vi "Event - Load Event Log.vi"(8 "error in":errorcluster) -> (0 "error out":errorcluster)   [LabVIEW 2019]
uses:
  Controls/Report - State.ctl
  Controls/Report - Data Structure.ctl
  <vilib>/httpClient/ClientHandle.ctl
  Controls/FGV States.ctl
  Controls/eFGV States.ctl
  Controls/JSON - Fileid.ctl
  <vilib>/httpClient/POSTBuffer.vi
  <vilib>/httpClient/LabVIEWHTTPClient.lvlib
panel:
  out "data":T1(array[cluster])
  in  "Tab Control":enum32{"Page 1", "Page 2"}(tab)
  in  "Listbox":i32(listbox)=-1 caption="Select Test"
  in  "Search":string
  in  "Generate":bool
  in  "Cancel":bool
  out "Total":u32
  in  "Pages":u32
  in  "Forward":bool
  in  "Back":bool
  in  "Event List":i32(listbox)
  in  "Back":bool
  # "of"
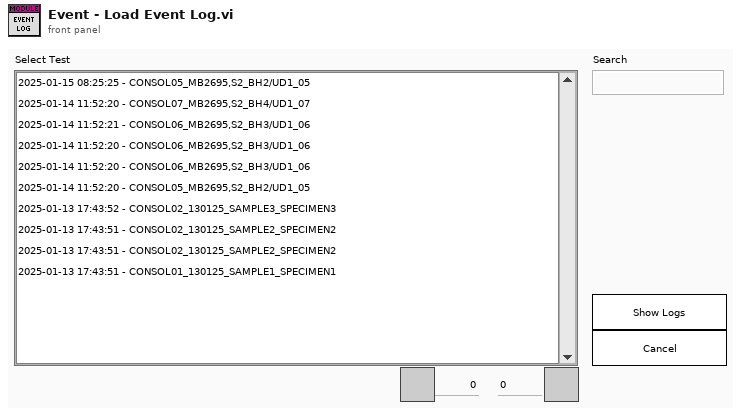
[diagram p1: front panel]
types:
  T1 = cluster{"id":string, "created_date":string, "testname":string, "jobno":string, "jobdesc":string, "sampleid":string, "date":string, "specimentno":string, "depth":string, "height":string, "diameter":string, "weight":string, "done":string}[]
  T2 = typedef "Report - State.ctl" = enum16{"Init", "Get File List", "Get Station Name", "Parse File List", "Idle", "Prepare to Generate", "Get Report", "Parse Report", "Get Data", "View T90", "Parse Data", "Convert to Excel", "Clean Up", "Close"}
  T3 = typedef "eFGV States.ctl" = enum16{"Init", "Read", "Write", "Exit"}
  T4 = typedef "FGV States.ctl" = enum16{"Read", "Write"}
  T5 = typedef "Report - Data Structure.ctl" = cluster{"API Ref":T6, "FileList":string[][], "Fileid":string, "testname":string[], "testtype":string[], "tdms":refnum<k34>, "TDMS Path":path, "tdms_path":string, "excel_path":string, "Excel Path":path, "List Name":string[], "Station Name":string[], "Plot":bool, "Tangent Point":string}
  T6 = typedef "LabVIEWHTTPClient.lvlib/ClientHandle.ctl" = refnum<k1>
  T7 = typedef "JSON - Fileid.ctl" = cluster{"status":string, "data":cluster{"id":string, "created_date":string, "testname":string, "jobno":string, "jobdesc":string, "sampleid":string, "date":string, "specimentno":string, "depth":string, "height":string, "diameter":string, "weight":string, "done":string}[]}
  T8 = cluster{"status":string, "data":cluster{"id":string, "created_date":string, "filename":string, "stage":string, "testplan":string, "station":string, "status":string, "delete":string}[]}
  T9 = cluster{"status":string, "data":cluster{"created_date":string, "message":string}[]}
  T10 = cluster{"id":string, "created_date":string, "filename":string, "stage":string, "testplan":string, "station":string, "status":string, "delete":string}[]
  T11 = cluster{"id":string, "created_date":string, "filename":string, "stage":string, "testplan":string, "station":string, "status":string, "delete":string}
  T12 = typedef "eventvkey.ctl" = enum16{"ASCII", "Enter", "Return", "Shift", "Ctrl", "Alt", "Cmd", "Opt", "Caps", "NumLock", "Clear", "Break", "Up", "Down", "Left", "Right", "Insert", "Delete", "Home", "End", "PageUp", "PageDown", "Escape", "Help", "Pause", "ScrollLock", "F1", "F2", "F3", "F4", "F5", "F6", "F7", "F8", "F9", "F10", "F11", "F12", "F13", "F14", "F15", "F16", "F17", "F18", "F19", "F20", "F21", "F22", "F23", "F24", "Play", "VolumeUp", "VolumeDown", "Mute", "Two Byte Char"}
  T13 = cluster{"created_date":string, "message":string}[]
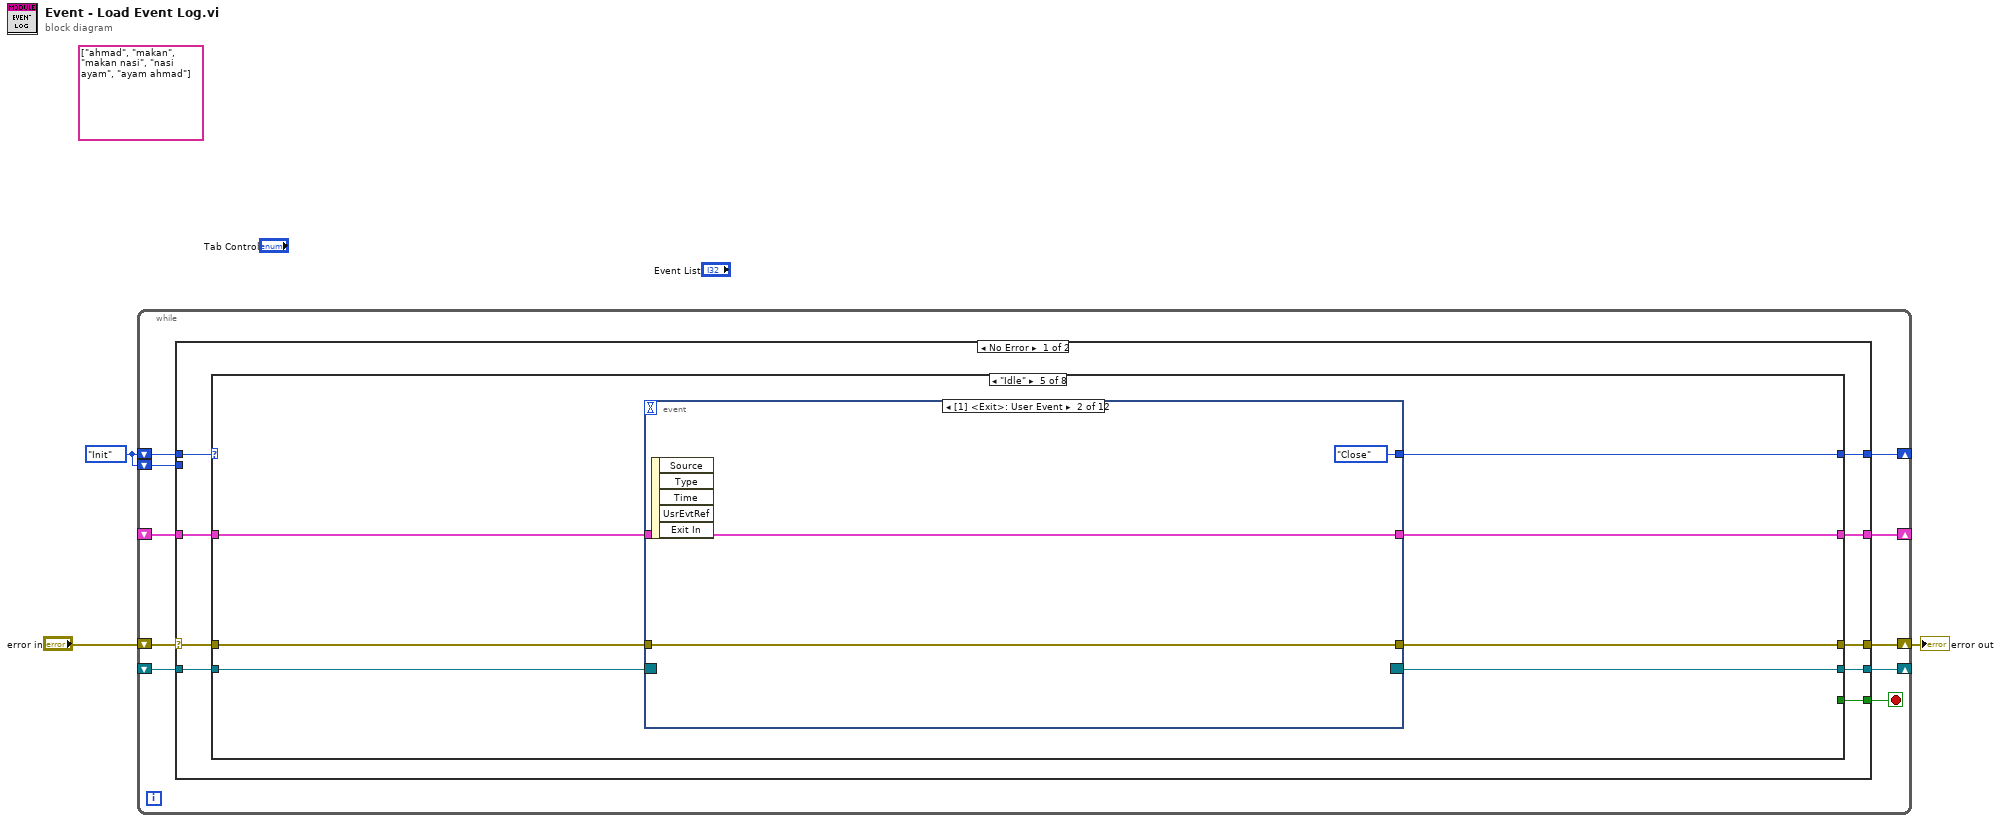
[diagram p0: block diagram]
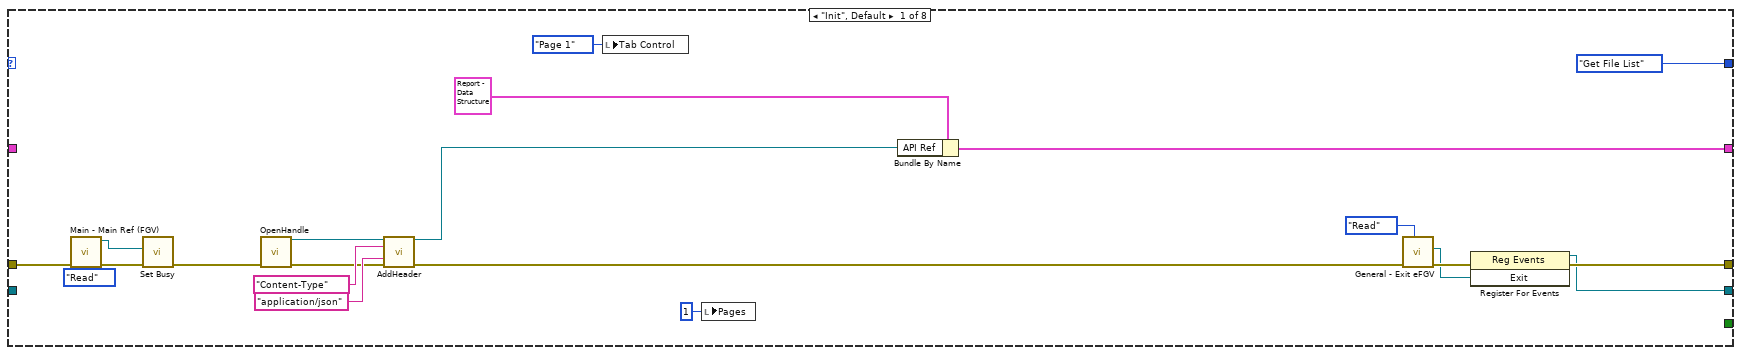
[diagram p2: hidden frame]
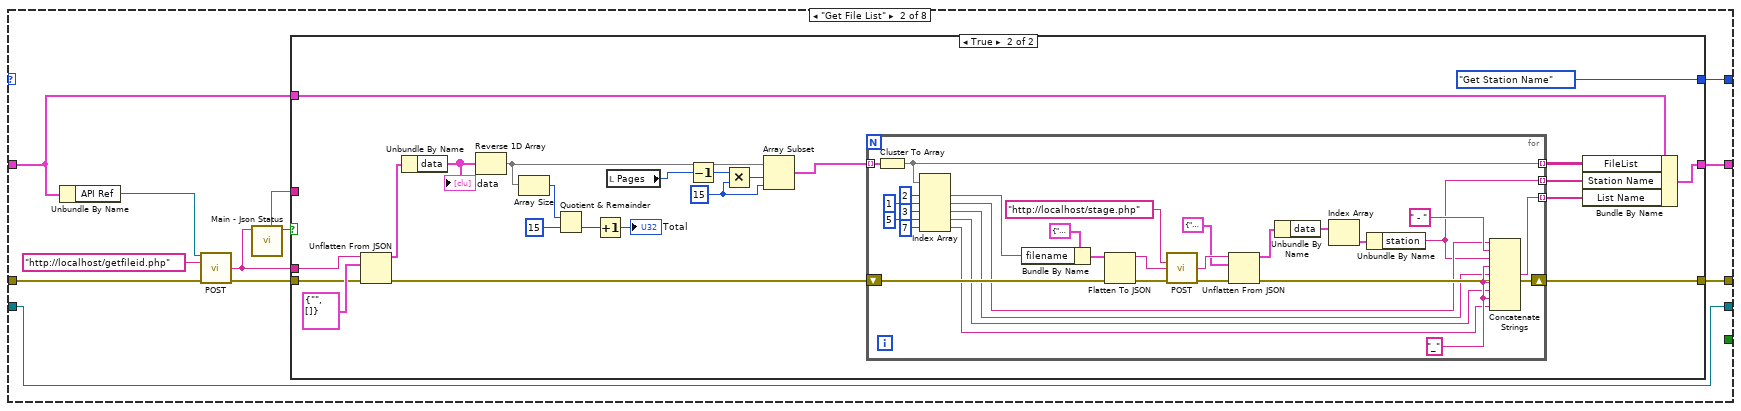
[diagram p3: hidden frame]
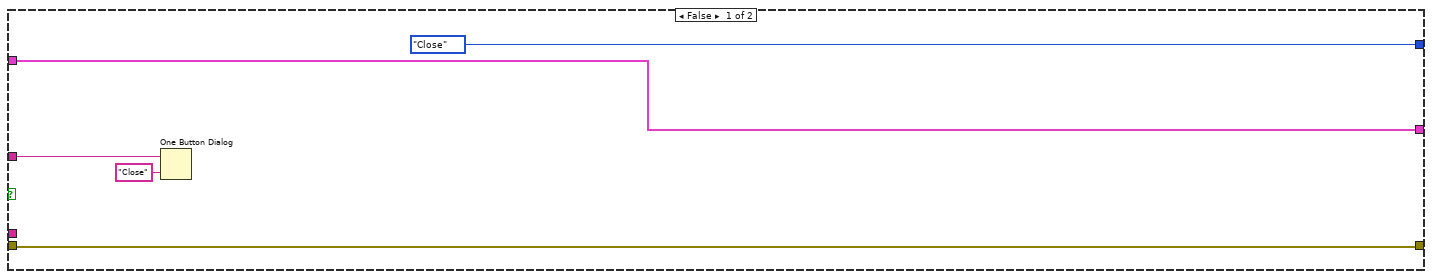
[diagram p4: hidden frame]
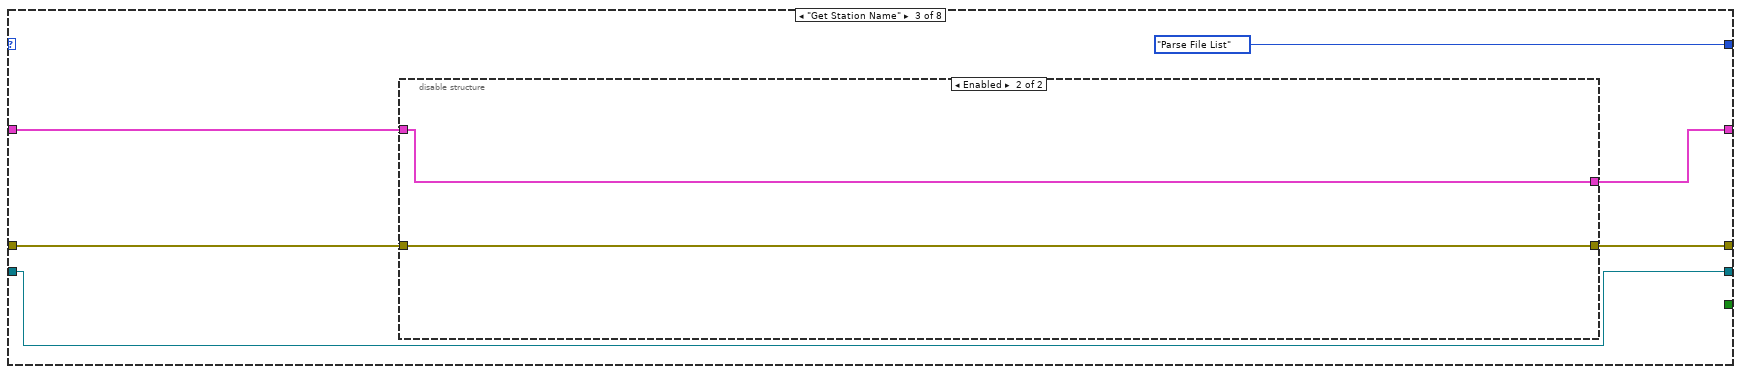
[diagram p5: hidden frame]
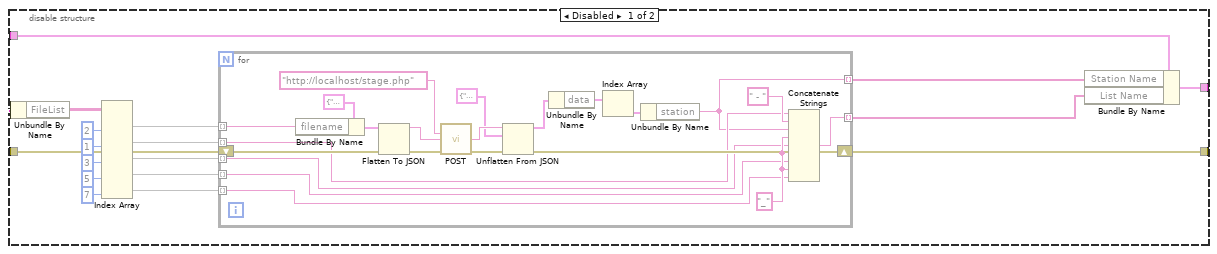
[diagram p6: hidden frame]
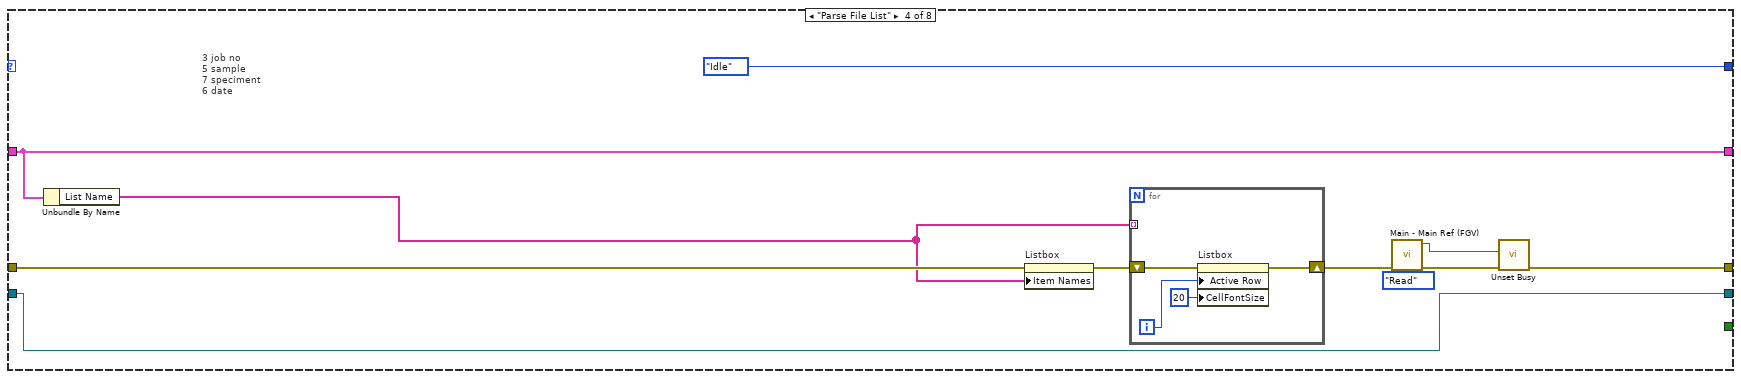
[diagram p7: hidden frame]
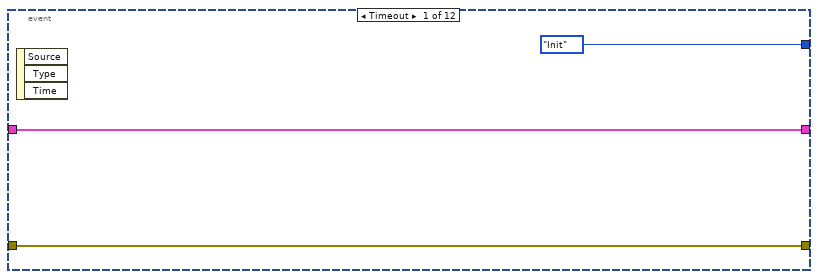
[diagram p8: hidden frame]
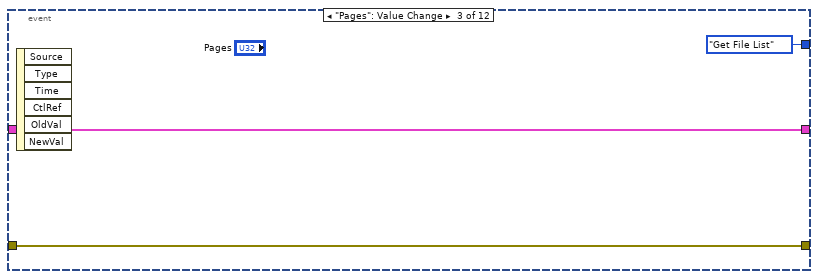
[diagram p9: hidden frame]
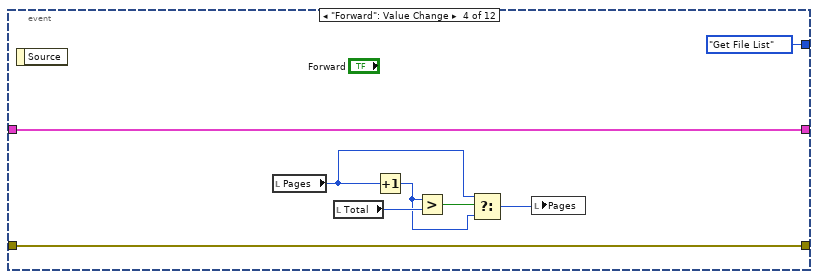
[diagram p10: hidden frame]
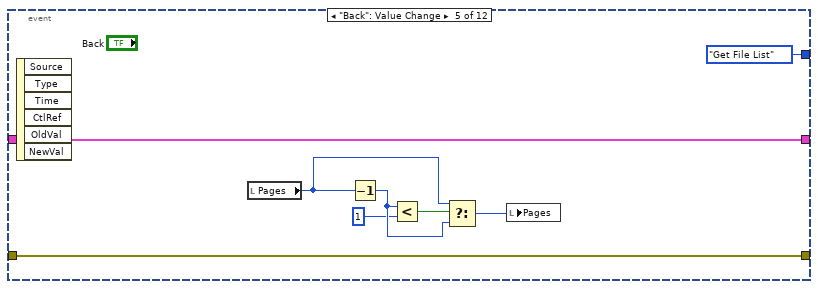
[diagram p11: hidden frame]
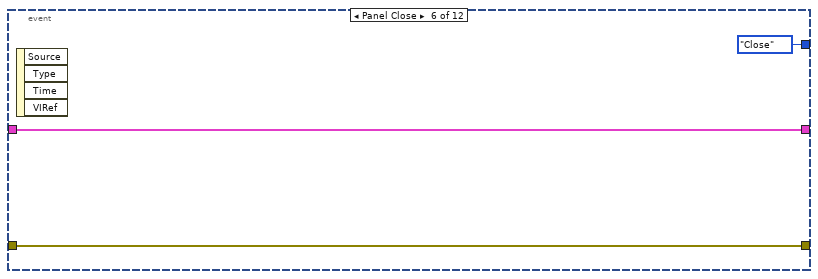
[diagram p12: hidden frame]
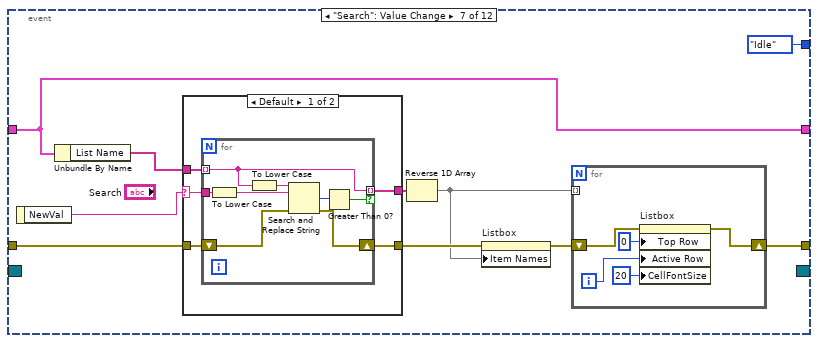
[diagram p13: hidden frame]
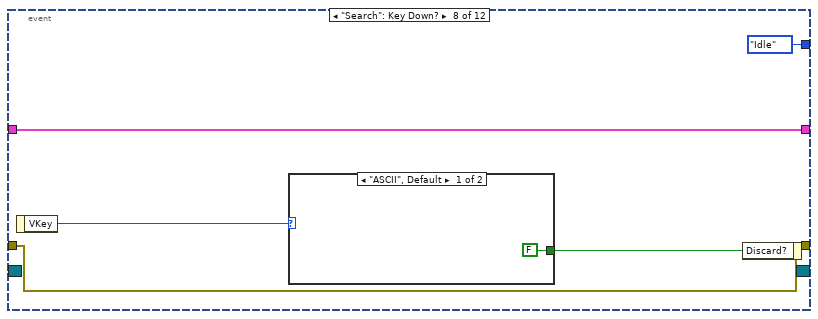
[diagram p15: hidden frame]
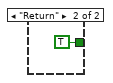
[diagram p16: hidden frame]
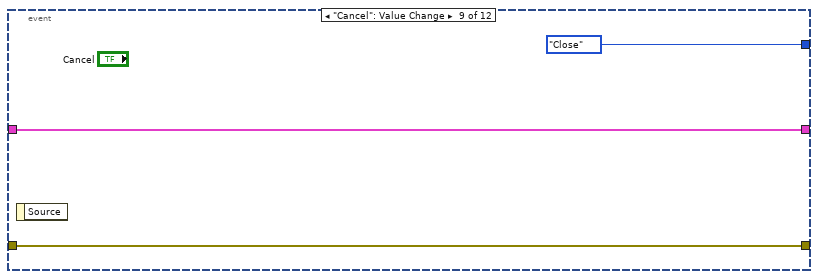
[diagram p17: hidden frame]
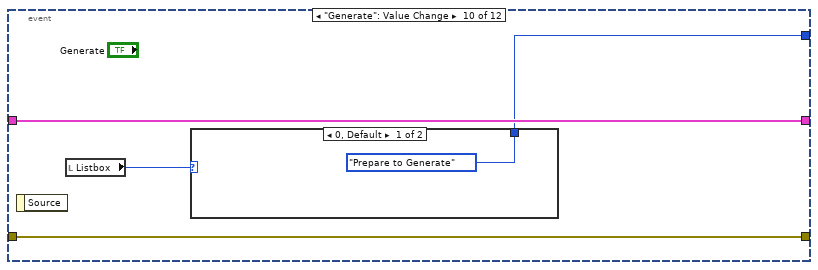
[diagram p18: hidden frame]
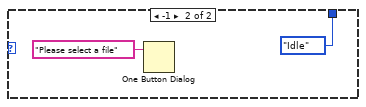
[diagram p19: hidden frame]
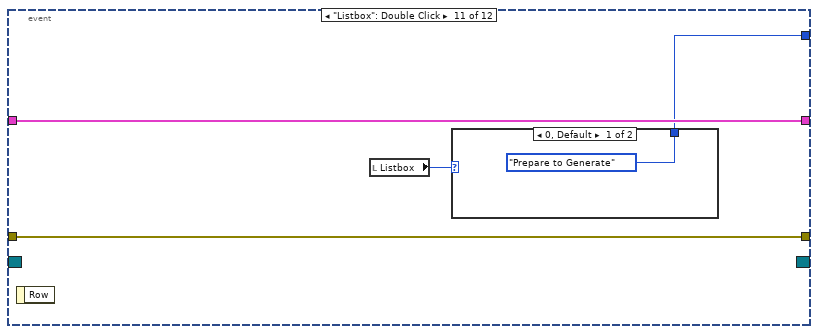
[diagram p20: hidden frame]
diagram:
  w1 = Report_-_State."Init"
  (unwired) string[] ["ahmad", "makan", "makan nasi", "nasi ayam", "ayam ahmad"]
  n1 = while {
    shift-right: [w10] -> w2
    shift-left: "error in" -> [w13]
    shift-right: [w11] -> _
    shift-left: w1 -> [w12]
    shift-right: [w9] -> _
    shift-left: _ -> [w8]
    shift-left: w1 -> [w6]
    shift-right: [w5] -> _
    shift-left: _ -> [w4]
    stop <- w7 stop-if-true
    n2 = case shown="No Error" w13 {
      selector: w13 -> [w20 w344]
      tunnel: w12 -> [w22 _]
      tunnel: [w21 Report_-_State."Close"] -> w11
      tunnel: [w19 w341] -> w10
      tunnel: [w18 w342] -> w9
      tunnel: w8 -> [w17 w342]
      tunnel: [w16 _] -> w7
      tunnel: w6 -> [_ w335]
      tunnel: [w15 w331] -> w5
      tunnel: w4 -> [w14 w331]
      frame No Error {
        n3 = case shown="\"Idle\"" w22 {
          tunnel: [Report_-_State."Get File List" ("f") w53 Report_-_State."Parse File List" Report_-_State."Idle" w179 Report_-_State."Get Report" Report_-_State."Idle" Report_-_State."Idle"] -> w21
          tunnel: w20 -> [w32 w54 w118 w169 w181 w271 w296 w327]
          tunnel: [w25 w51 w117 w163 w180 w285 w308 w324] -> w19
          tunnel: [w37 w48 w115 w167 w177 w276 w313 T5 {"API Ref"=refnum, "FileList"=[], "Fileid"="", "testname"=[], "testtype"=[], "tdms"=refnum, "TDMS Path"=path "", "tdms_path"="", "excel_path"="", "Excel Path"=path "", "List Name"=[], "Station Name"=[], "Plot"=FALSE, "Tangent Point"=""}] -> w18
          tunnel: w17 -> [_ w49 w114 w167 w178 w275 w313 w326]
          tunnel: [_ _ _ _ _ _ _ TRUE] -> w16
          tunnel: [w23 w44 w113 w160 w175 w268 w287 w321] -> w15
          tunnel: w14 -> [_ w44 w113 w160 w176 w268 w287 w321]
          frame "Init", Default {
            n4 = call "Main - Main Ref (FGV).vi"("Action"=FGV_States."Read", "error in"=w32) -> ("error out"=w33:errorcluster, "This VI out"=w31:refnum<vi>)  [unwired: 8 in]
            n5 = call <vilib>:"Set Busy.vi"("error in (no error)"=w33, "VI reference (current VI)"=w31) -> ("error out"=w35:errorcluster)  [unwired: 8 in, 1 out]
            n6 = call <vilib>:"OpenHandle.vi"("error in (no error)"=w35) -> ("client handle out"=w41:T6, "error out"=w40:errorcluster)  [unwired: 13 in]
            n7 = call <vilib>:"AddHeader.vi"("client handle"=w41, "header"="Content-Type", "value"="application/json", "error in (no error)"=w40) -> ("client handle out"=w38:T6, "error out"=w28:errorcluster)  [unwired: 10 in]
            n8 = local write "Tab Control"(enum32{"Page 1", "Page 2"}."Page 1" ("Tab Control")) -> ()
            n9 = local write "Pages"(u32 1 ("Pages")) -> ()
            n10 = Bundle By Name(cluster=T5 {"API Ref"=refnum, "FileList"=[], "Fileid"="", "testname"=[], "testtype"=[], "tdms"=refnum, "TDMS Path"=path "", "tdms_path"="", "excel_path"="", "Excel Path"=path "", "List Name"=[], "Station Name"=[], "Plot"=FALSE, "Tangent Point"=""}, "API Ref"=w38) -> (w37:T5)
            n11 = call "General - Exit eFGV.vi"("eFGV States"=eFGV_States."Read", "error in (no error)"=w28) -> ("error out"=w27:errorcluster, "Exit"=w24:refnum<user-event>)  [unwired: 7 in, 1 out]
            n12 = register-events(error in=w27, w24) -> (reference out=w23:refnum<event-registration>, error out=w25:errorcluster)  [unwired: 1 in]
          }
          frame "Get File List" {
            n13 = Unbundle By Name(w49) -> ("API Ref"=w50:T6)
            n14 = call-poly <vilib>:"POST.vi"("client handle"=w50, "url"="http://localhost/getfileid.php", "error in (no error)"=w54) -> ("body"=w47:string, "error out"=w52:errorcluster)  [unwired: 9 in, 2 out]
            n15 = call "Main - Json Status.vi"("json"=w47) -> ("Success?"=w46:bool, "message"=w45:string)  [unwired: 9 in]
            n16 = case shown="True" w46 {
              tunnel: [Report_-_State."Close" Report_-_State."Get Station Name"] -> w53
              tunnel: w52 -> [w57 w81]
              tunnel: [w57 w74] -> w51
              tunnel: w47 -> [_ w80]
              tunnel: w49 -> [w59 w77]
              tunnel: [w59 w75] -> w48
              tunnel: w45 -> [w58 _]
              frame False {
                n17 = One Button Dialog(message=w58, button name ("OK")="Close") -> ()  [unwired: 1 out]
              }
              frame True {
                w67 = 15 ("length")
                n18 = Unflatten From JSON(JSON string=w80, type and defaults=T7 {"status"="", "data"=[]}, error in (no error)=w81) -> (value=w78:T7, error out=w62:errorcluster)  [unwired: 4 in]
                n19 = Unbundle By Name(w78) -> ("data"=w79:T1)
                "data" <- w79
                n20 = Reverse 1D Array(array=w79) -> (reversed array=w66:T1)
                n21 = Array Size(array=w66) -> (size(s)=w70:i32)
                n22 = Quotient & Remainder(x=w70, y=15) -> (floor(x/y)=w71:i32)  [unwired: 1 out]
                n23 = Increment(x=w71) -> (x+1=→"Total":i32)
                n24 = local read "Pages"() -> (w63:u32)
                n25 = Decrement(x=w63) -> (x-1=w64:u32)
                n26 = Multiply(x=w64, y=w67) -> (x*y=w68:u32)
                n27 = Array Subset(array=w66, index=w68, length=w67) -> (w65:T1)
                n28 = for {
                  tunnel: w65 -> [w112] mode=indexing
                  tunnel: [w111] -> w76 mode=indexing
                  shift-right: [w91] -> w74
                  shift-left: w62 -> [w92]
                  tunnel: [w85] -> w72 mode=indexing
                  tunnel: [w84] -> w73 mode=indexing
                  w96 = "_" ("string")
                  n29 = Cluster To Array(cluster=w112) -> (array=w111:string[])
                  n30 = Index Array(array=w111, index #1=2 ("disabled index (col)"), index #2=1 ("index (col)"), index #3=3 ("index (col)"), index #4=5 ("index (col)"), index #5=7 ("index (col)")) -> (element #1=w90:string, element #2=w89:string, element #3=w88:string, element #4=w87:string, element #5=w86:string)
                  n31 = Bundle By Name(cluster=cluster{"action":string, "filename":string} {"action"="read", "filename"=""}, "filename"=w90) -> (w101:cluster{"action":string, "filename":string})
                  n32 = Flatten To JSON(anything=w101, error in (no error)=w92) -> (JSON string=w102:string, 11:w105:errorcluster)  [unwired: 1 in]
                  n33 = call-poly <vilib>:"POST.vi"("url"="http://localhost/stage.php", "buffer"=w102, "error in (no error)"=w105) -> ("body"=w103:string, "error out"=w104:errorcluster)  [unwired: 9 in, 2 out]
                  n34 = Unflatten From JSON(JSON string=w103, type and defaults=T8 {"status"="read", "data"=[]} ("Cluster"), error in (no error)=w104) -> (value=w100:T8, error out=w91:errorcluster)  [unwired: 4 in]
                  n35 = Unbundle By Name(w100) -> ("data"=w99:T10)
                  n36 = Index Array(array=w99) -> (element=w98:T11)  [unwired: 1 in]
                  n37 = Unbundle By Name(w98) -> ("station"=w84:string)
                  n38 = Concatenate Strings(w89, " - " ("string"), w84, w96, w88, w96, w87, w96, w86) -> (w85:string)
                }
                n39 = Bundle By Name(cluster=w77, "FileList"=w76, "Station Name"=w73, "List Name"=w72) -> (w75:T5)
              }
            }
          }
          frame "Get Station Name" {
            n40 = disable-structure shown="Enabled" {
              disable-tunnel: w118 -> [w135 w158]
              disable-tunnel: [w134 w158] -> w117
              disable-tunnel: [w129 w159] -> w115
              disable-tunnel: w114 -> [w128 w159]
              frame Disabled {
                n41 = Unbundle By Name(w128) -> ("FileList"=w133:string[][])
                n42 = Index Array(array=w133, index (col) #1=2 ("disabled index (col)"), index (col) #2=1 ("index (col)"), index (col) #3=3 ("index (col)"), index (col) #4=5 ("index (col)"), index (col) #5=7 ("index (col)")) -> (element #1=w131:string[], element #2=w123:string[], element #3=w122:string[], element #4=w121:string[], element #5=w120:string[])  [unwired: 5 in]
                n43 = for {
                  shift-right: [w150] -> w134
                  shift-left: w135 -> [w151]
                  tunnel: w131 -> [w147] mode=indexing
                  tunnel: [w140] -> w130 mode=indexing
                  tunnel: w123 -> [w141] mode=indexing
                  tunnel: w122 -> [w139] mode=indexing
                  tunnel: w121 -> [w138] mode=indexing
                  tunnel: w120 -> [w137] mode=indexing
                  tunnel: [w136] -> w119 mode=indexing
                  w142 = "_" ("string")
                  n44 = Bundle By Name(cluster=cluster{"action":string, "filename":string} {"action"="read", "filename"=""}, "filename"=w147) -> (w148:cluster{"action":string, "filename":string})
                  n45 = Flatten To JSON(anything=w148, error in (no error)=w151) -> (JSON string=w154:string, 11:w157:errorcluster)  [unwired: 1 in]
                  n46 = call-poly <vilib>:"POST.vi"("url"="http://localhost/stage.php", "buffer"=w154, "error in (no error)"=w157) -> ("body"=w155:string, "error out"=w156:errorcluster)  [unwired: 9 in, 2 out]
                  n47 = Unflatten From JSON(JSON string=w155, type and defaults=T8 {"status"="read", "data"=[]} ("Cluster"), error in (no error)=w156) -> (value=w146:T8, error out=w150:errorcluster)  [unwired: 4 in]
                  n48 = Unbundle By Name(w146) -> ("data"=w145:T10)
                  n49 = Index Array(array=w145) -> (element=w144:T11)  [unwired: 1 in]
                  n50 = Unbundle By Name(w144) -> ("station"=w140:string)
                  n51 = Concatenate Strings(w141, " - " ("string"), w140, w142, w139, w142, w138, w142, w137) -> (w136:string)
                }
                n52 = Bundle By Name(cluster=w128, "Station Name"=w130, "List Name"=w119) -> (w129:T5)
              }
              frame Enabled {
              }
            }
          }
          frame "Parse File List" {
            # "3 job no\n5 sample\n7 speciment\n6 date"
            n53 = Unbundle By Name(w167) -> ("List Name"=w161:string[])
            n54 = property on="Listbox" class="LstBox (strict)"(error in=w169, "Item Names"=w161) -> (error out=w168:errorcluster)  [unwired: 1 in, 1 out]
            n55 = for {
              shift-right: [w172] -> w165
              shift-left: w168 -> [w173]
              tunnel: w161 -> [_] mode=indexing
              i -> [w171]
              n56 = property on="Listbox" class="LstBox (strict)"(error in=w173, "Active Row"=w171, "CellFontSize"=u32 20 ("Active Row:Cell Font:Size")) -> (error out=w172:errorcluster)  [unwired: 1 in, 1 out]
            }
            n57 = call "Main - Main Ref (FGV).vi"("Action"=FGV_States."Read", "error in"=w165) -> ("error out"=w164:errorcluster, "This VI out"=w162:refnum<vi>)  [unwired: 8 in]
            n58 = call <vilib>:"Unset Busy.vi"("error in (no error)"=w164, "VI reference (current VI)"=w162) -> ("error out"=w163:errorcluster)  [unwired: 9 in]
          }
          frame "Idle" {
            n59 = event shown="[1] <Exit>: User Event" {
              selector: w176 -> [_ _ _ _ _ _ _ _ _ _ _ _]
              dyn-events: [_ _ _ _ _ _ _ _ _ _ _ _] -> w175
              timeout: _ -> [_ _ _ _ _ _ _ _ _ _ _ _]
              tunnel: w181 -> [w184 w187 w188 w196 w206 w207 w215 w240 w248 w252 w258 w267]
              tunnel: [w184 w187 w188 w196 w206 w207 w214 w240 w248 w252 w258 w267] -> w180
              tunnel: [Report_-_State."Init" Report_-_State."Close" ("f") Report_-_State."Get File List" ("f") Report_-_State."Get File List" ("f") Report_-_State."Get File List" ("f") Report_-_State."Close" Report_-_State."Idle" Report_-_State."Idle" ("f") Report_-_State."Close" w250 w257 Report_-_State."Idle" ("f")] -> w179
              tunnel: w178 -> [w182 w186 w190 w197 w205 w208 w212 w244 w249 w253 w260 w266]
              tunnel: [w182 w186 w190 w197 w205 w208 w212 w244 w249 w253 w260 w266] -> w177
              event Timeout {
                n60 = event-data() -> ()  [unwired: 1 in, 3 out]
              }
              event User Event {
                n61 = event-data() -> ()  [unwired: 1 in, 5 out]
              }
              event "Pages": Value Change {
                n62 = event-data() -> ()  [unwired: 1 in, 6 out]
              }
              event "Forward": Value Change {
                n63 = event-data() -> ()  [unwired: 1 in, 1 out]
                n64 = local read "Pages"() -> (w193:u32)
                n65 = local read "Total"() -> (w195:u32)
                n66 = Increment(x=w193) -> (x+1=w192:u32)
                n67 = Greater?(x=w192, y=w195) -> (0:w194:bool)
                n68 = Select(t=w193, s=w194, f=w192) -> (s? t:f=w191:u32)
                n69 = local write "Pages"(w191) -> ()
              }
              event "Back": Value Change {
                n70 = event-data() -> ()  [unwired: 1 in, 6 out]
                n71 = local read "Pages"() -> (w202:u32)
                n72 = Decrement(x=w202) -> (x-1=w201:u32)
                n73 = Less?(x=w201, y=u32 1) -> (x < y?=w203:bool)
                n74 = Select(t=w202, s=w203, f=w201) -> (s? t:f=w200:u32)
                n75 = local write "Pages"(w200) -> ()
              }
              event Panel Close {
                n76 = event-data() -> ()  [unwired: 1 in, 4 out]
              }
              event "Search": Value Change {
                n77 = event-data() -> ("NewVal"=w213:string)  [unwired: 1 in]
                n78 = Unbundle By Name(w212) -> ("List Name"=w210:string[])
                n79 = case shown="Default" w213 {
                  selector: w213 -> [w225 _]
                  tunnel: w210 -> [w229 w239]
                  tunnel: w215 -> [w228 w238]
                  tunnel: [w227 w238] -> w218
                  tunnel: [w226 w239] -> w216
                  frame Default {
                    n80 = for {
                      tunnel: w225 -> [w237]
                      tunnel: [w234] -> w226 mode=indexing if=w235
                      tunnel: w229 -> [w234] mode=indexing
                      shift-right: [w232] -> w227
                      shift-left: w228 -> [w233]
                      n81 = To Lower Case(string=w237) -> (all lower case string=w231:string)
                      n82 = To Lower Case(string=w234) -> (all lower case string=w230:string)
                      n83 = Search and Replace String(input string=w230, search string=w231, error in=w233) -> (number of replacements=w236:i32, error out=w232:errorcluster)  [unwired: 5 in, 2 out]
                      n84 = Greater Than 0?(x=w236) -> (x > 0?=w235:bool)
                    }
                  }
                  frame "" {
                  }
                }
                n85 = Reverse 1D Array(array=w216) -> (reversed array=w211:string[])
                n86 = property on="Listbox" class="LstBox (strict)"(error in=w218, "Item Names"=w211) -> (error out=w217:errorcluster)  [unwired: 1 in, 1 out]
                n87 = for {
                  shift-right: [w222] -> w214
                  shift-left: w217 -> [w223]
                  tunnel: w211 -> [_] mode=indexing
                  i -> [w221]
                  n88 = property on="Listbox" class="LstBox (strict)"(error in=w223, "Top Row"=0, "Active Row"=w221, "CellFontSize"=u32 20 ("Active Row:Cell Font:Size")) -> (error out=w222:errorcluster)  [unwired: 1 in, 1 out]
                }
              }
              event "Search": Key Down? {
                n89 = event-data() -> ("VKey"=w242:T12)  [unwired: 1 in]
                n90 = case shown="\"ASCII\", Default" w242 {
                  tunnel: [FALSE TRUE] -> w241
                  frame "ASCII", Default {
                  }
                  frame "Return" {
                  }
                }
                n91 = event-data("Discard?"=w241) -> ()  [unwired: 1 in, 1 out]
              }
              event "Cancel": Value Change {
                n92 = event-data() -> ()  [unwired: 1 in, 1 out]
              }
              event "Generate": Value Change {
                n93 = event-data() -> ()  [unwired: 1 in, 1 out]
                n94 = local read "Listbox"() -> (w251:i32)
                n95 = case shown="0, Default" w251 {
                  tunnel: [Report_-_State."Prepare to Generate" Report_-_State."Idle"] -> w250
                  frame 0, Default {
                  }
                  frame -1 {
                    n96 = One Button Dialog(message="Please select a file") -> ()  [unwired: 1 in, 1 out]
                  }
                }
              }
              event "Listbox": Double Click {
                n97 = event-data() -> ()  [unwired: 1 in, 1 out]
                n98 = local read "Listbox"() -> (w259:i32)
                n99 = case shown="0, Default" w259 {
                  tunnel: [Report_-_State."Prepare to Generate" Report_-_State."Idle"] -> w257
                  frame 0, Default {
                  }
                  frame -1 {
                    n100 = One Button Dialog(message="Please select a file") -> ()  [unwired: 1 in, 1 out]
                  }
                }
              }
              event "Back": Value Change {
                n101 = event-data() -> ()  [unwired: 1 in, 1 out]
                n102 = local write "Tab Control"(enum32{"Page 1", "Page 2"}."Page 1" ("Tab Control")) -> ()
              }
            }
          }
          frame "Prepare to Generate" {
            n103 = call "Main - Main Ref (FGV).vi"("Action"=FGV_States."Read", "error in"=w271) -> ("error out"=w272:errorcluster, "This VI out"=w270:refnum<vi>)  [unwired: 8 in]
            n104 = call <vilib>:"Set Busy.vi"("error in (no error)"=w272, "VI reference (current VI)"=w270) -> ("error out"=w274:errorcluster)  [unwired: 8 in, 1 out]
            n105 = property on="Listbox" class="LstBox (strict)"(error in=w274) -> (error out=w285:errorcluster, "Item Names"=w283:string[])  [unwired: 1 in, 1 out]
            n106 = Unbundle By Name(w275) -> ("FileList"=w282:string[][], "List Name"=w269:string[])
            n107 = Index Array(array=w282, index (col)=0 ("disabled index (col)")) -> (element=w279:string[])  [unwired: 1 in]
            n108 = Index Array(array=w283, index="Listbox") -> (element=w280:string)
            n109 = Search 1D Array(1D array=w269, element=w280) -> (index of element=w278:i32)  [unwired: 1 in]
            n110 = Index Array(array=w279, index=w278) -> (element=w277:string)
            n111 = Bundle By Name(cluster=w275, "Fileid"=w277) -> (w276:T5)
          }
          frame "Get Report" {
            n112 = Unbundle By Name(w313) -> ("Fileid"=w294:string, "API Ref"=w293:T6)
            n113 = local write "Tab Control"(enum32{"Page 1", "Page 2"}."Page 2" ("Tab Control")) -> ()
            n114 = Bundle By Name(cluster=cluster{"action":string, "fileid":string} {"action"="read", "fileid"=""}, "action"="read", "fileid"=w294) -> (w297:cluster{"action":string, "fileid":string})
            n115 = Flatten To JSON(anything=w297, error in (no error)=w296) -> (JSON string=w304:string, 11:w305:errorcluster)  [unwired: 1 in]
            n116 = call-poly <vilib>:"POST.vi"("client handle"=w293, "url"="http://localhost/allevent.php", "buffer"=w304, "error in (no error)"=w305) -> ("body"=w307:string, "error out"=w303:errorcluster)  [unwired: 8 in, 2 out]
            n117 = Unflatten From JSON(JSON string=w307, type and defaults=T9 {"status"="read", "data"=[]}, error in (no error)=w303) -> (value=w301:T9, error out=w292:errorcluster)  [unwired: 4 in]
            n118 = Unbundle By Name(w301) -> ("data"=w300:T13)
            n119 = Reverse 1D Array(array=w300) -> (reversed array=w299:T13)
            n120 = for {
              tunnel: w299 -> [w320] mode=indexing
              tunnel: [w316] -> w290
              tunnel: w292 -> [w316]
              tunnel: [w315] -> w289 mode=indexing
              n121 = Unbundle By Name(w320) -> ("created_date"=w319:string, "message"=w318:string)
              n122 = Concatenate Strings(w319, "    :    " ("string"), w318) -> (w315:string)
            }
            n123 = property on="Event List" class="LstBox (strict)"(error in=w290, "Item Names"=w289, "Value"=-1 ("Active Row:Active Row Number")) -> (error out=w291:errorcluster)  [unwired: 1 in, 1 out]
            n124 = call "Main - Main Ref (FGV).vi"("Action"=FGV_States."Read", "error in"=w291) -> ("error out"=w310:errorcluster, "This VI out"=w309:refnum<vi>)  [unwired: 8 in]
            n125 = call <vilib>:"Unset Busy.vi"("error in (no error)"=w310, "VI reference (current VI)"=w309) -> ("error out"=w308:errorcluster)  [unwired: 9 in]
          }
          frame "Close" {
            n126 = Unbundle By Name(w326) -> ("API Ref"=w325:T6)
            n127 = call <vilib>:"CloseHandle.vi"("client handle"=w325, "error in (no error)"=w327) -> ("error out"=w322:errorcluster)  [unwired: 13 in]
            n128 = control-ref of="This VI"() -> (w323:refnum<vi>)
            n129 = invoke class="VI" method="FP.Close"(reference=w323, error in=w322) -> (error out=w324:errorcluster)  [unwired: 1 in, 2 out]
          }
        }
      }
      frame Error {
        n130 = Unbundle By Name(w344) -> ("source"=w338:string)
        n131 = call <vilib>:"Clear Errors.vi"("error in (no error)"=w344) -> ("error out"=w337:errorcluster)  [unwired: 5 in, 1 out]
        n132 = Format Into String(error in=w337, w335) -> (resulting string=w332:string, error out=w336:errorcluster)  [unwired: 2 in]
        n133 = Concatenate Strings(w338, "\n" ("string"), w332) -> (w334:string)
        n134 = call "Main - Main Ref (FGV).vi"("Action"=FGV_States."Read", "error in"=w336) -> ("error out"=w346:errorcluster, "This VI out"=w345:refnum<vi>)  [unwired: 8 in]
        n135 = call <vilib>:"Unset Busy.vi"("error in (no error)"=w346, "VI reference (current VI)"=w345) -> ("error out"=w343:errorcluster)  [unwired: 9 in]
        n136 = flat-sequence {
          tunnel: w334 -> [w351]
          tunnel: [w350] -> w340
          tunnel: w343 -> [w350]
          frame #0 {
            n137 = One Button Dialog(message=w351) -> ()  [unwired: 1 in, 1 out]
          }
        }
        n138 = Unbundle By Name(w342) -> ("API Ref"=w339:T6)
        n139 = call <vilib>:"CloseHandle.vi"("client handle"=w339, "error in (no error)"=w340) -> ("error out"=w341:errorcluster)  [unwired: 13 in]
        n140 = Wait (ms)(milliseconds to wait=u32 1000) -> ()  [unwired: 1 out]
      }
    }
  }
  "error out" <- w2
